vi "YKMW100 Check Modules.vi"(8 "Error In":errorcluster, 10 "Check Module Input":string, 11 "Input Modules (Out of Order)":string[](array[string])) -> (0 "Error Out":errorcluster, 3 "Input Modules (In Order)":string[](array[string]))   [LabVIEW 2016]
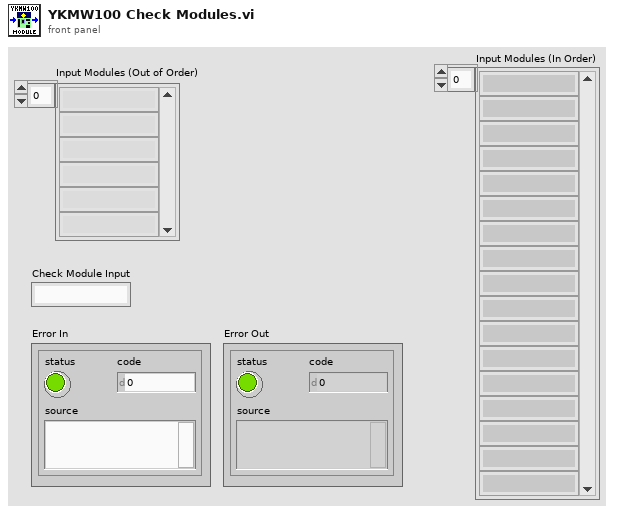
[diagram p1: front panel]
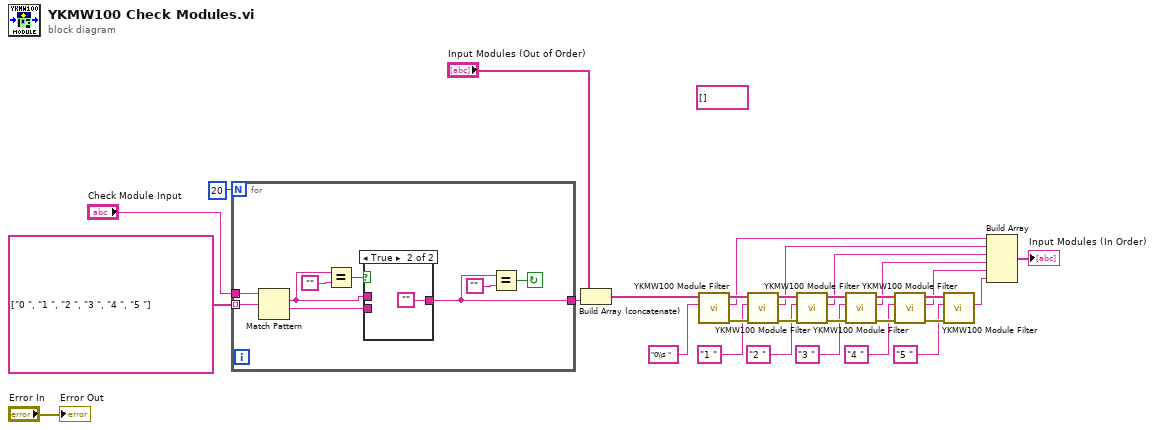
[diagram p0: block diagram]
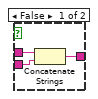
[diagram p2: hidden frame]
diagram:
  (unwired) string[] []
  n1 = for {
    N: 20 -> [_]
    tunnel: "Check Module Input" -> [w39]
    tunnel: string[] ["0 ", "1 ", "2 ", "3 ", "4 ", "5 "] ("Read Array 2") -> [w38] mode=indexing
    tunnel: [w31] -> w25
    stop <- w32 continue-if-true
    n2 = Match Pattern(string=w39, regular expression=w38) -> (match substring=w35:string, after substring=w34:string)  [unwired: 1 in, 2 out]
    n3 = Equal?(x=w35, y="") -> (x = y?=w36:bool)
    n4 = case shown="True" w36 {
      tunnel: w35 -> [w42 _]
      tunnel: w34 -> [w41 _]
      tunnel: [w40 ""] -> w31
      frame False {
        n5 = Concatenate Strings(w42, w41) -> (w40:string)
      }
      frame True {
      }
    }
    n6 = Equal?(x=w31, y="") -> (x = y?=w32:bool)
  }
  n7 = Build Array (concatenate)("Input Modules (Out of Order)", w25) -> (w24:string[])
  n8 = call "YKMW100 Module Filter.vi"("Select Module"="0\\s ", "All Data Input"=w24) -> ("Error Out"=w21:errorcluster, "Specific Point"=w6:string, "All Data Output"=w16:string[])  [unwired: 7 in]
  n9 = call "YKMW100 Module Filter.vi"("Error In"=w21, "Select Module"="1 " ("Read Buffer"), "All Data Input"=w16) -> ("Error Out"=w20:errorcluster, "Specific Point"=w5:string, "All Data Output"=w15:string[])  [unwired: 6 in]
  n10 = call "YKMW100 Module Filter.vi"("Error In"=w20, "Select Module"="2 " ("Read Buffer"), "All Data Input"=w15) -> ("Error Out"=w19:errorcluster, "Specific Point"=w4:string, "All Data Output"=w14:string[])  [unwired: 6 in]
  n11 = call "YKMW100 Module Filter.vi"("Error In"=w19, "Select Module"="3 " ("Read Buffer"), "All Data Input"=w14) -> ("Error Out"=w18:errorcluster, "Specific Point"=w3:string, "All Data Output"=w13:string[])  [unwired: 6 in]
  n12 = call "YKMW100 Module Filter.vi"("Error In"=w18, "Select Module"="4 " ("Read Buffer"), "All Data Input"=w13) -> ("Error Out"=w17:errorcluster, "Specific Point"=w2:string, "All Data Output"=w12:string[])  [unwired: 6 in]
  n13 = call "YKMW100 Module Filter.vi"("Error In"=w17, "Select Module"="5 " ("Read Buffer"), "All Data Input"=w12) -> ("Specific Point"=w1:string)  [unwired: 6 in, 2 out]
  n14 = Build Array(w6, w5, w4, w3, w2, w1) -> (→"Input Modules (In Order)":string[])
  "Error Out" <- "Error In"
